vi "Transverse Triangulation Function.vi"(9 "output selector":T1, 10 "data":T2, 11 "X":dbl[](array[numeric])) -> (0 "error out":errorcluster, 1 "inequality constraint function values":dbl[](array[numeric]), 2 "equality constraint function values":dbl[](array[numeric]), 3 "objective function value":dbl)   [LabVIEW 2012]
doc: "This template is the starting point for creating an objective function, equality constraint function and inequality constraint function to be passed to the Constrained Nonlinear Optimization.vi."
uses:
  <vilib>/gmath/NumericalOptimization/objective function data.ctl
  <vilib>/gmath/NumericalOptimization/cno_output select.ctl
  <vilib>/gmath/NI_Gmath.lvlib
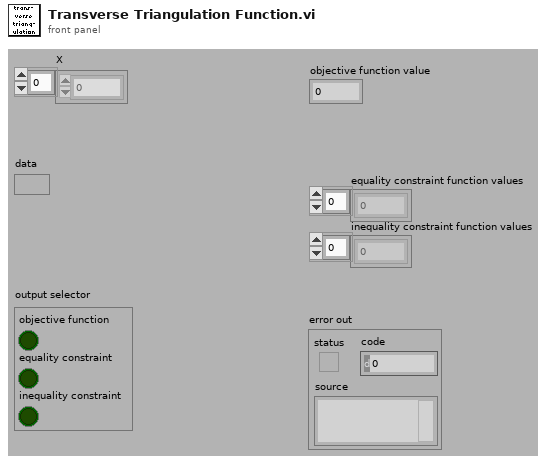
[diagram p1: front panel]
types:
  T1 = typedef "NI_Gmath.lvlib/cno_output select.ctl" = cluster{"objective function":bool, "equality constraint":bool, "inequality constraint":bool}
  T2 = typedef "NI_Gmath.lvlib/objective function data.ctl" = variant
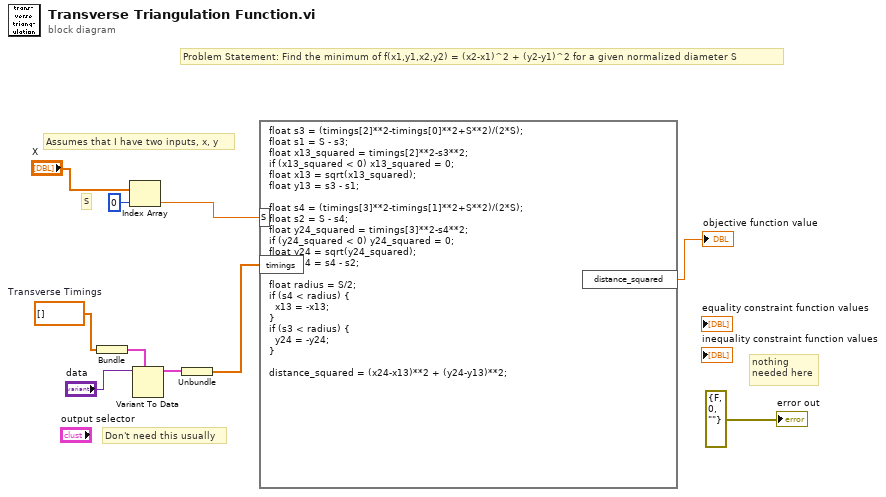
[diagram p0: block diagram]
diagram:
  w7 = dbl[] []  # Transverse Timings
  # "nothing \nneeded here"
  # "S"
  # "Problem Statement: Find the minimum of f(x1,y1,x2,y2) = (x2-x1)^2 + (y2-y1)^2 for a given normalized diameter S"
  # "Don't need this usually"
  # "Assumes that I have two inputs, x, y"
  n1 = Bundle("Transverse Timings"=w7) -> (w5:cluster{"Transverse Timings":dbl[]})  [unwired: 1 in]
  n2 = Index Array(array="X", index=0) -> (element=w2:dbl)
  n3 = Variant To Data(type=w5, Variant="data") -> (data=w4:cluster{"Transverse Timings":dbl[]})  [unwired: 1 in, 1 out]
  n4 = Unbundle(w4) -> ("Transverse Timings"=w3:dbl[])
  n5 = formula code="float s3 = (timings[2]**2-timings[0]**2+S**2)/(2*S);\nfloat s1 = S - s3;\nfloat x13_squared = timings[2]**2-s3**2;\nif (x13_squared < 0) x13_squared = 0;\nfloat x13 = sqrt(x13_squared);\nfloat y13 = s3 - s1;\n\nfloat s4 = (timings[3]**2-timings[1]**2+S**2)/(2*S);\nfloat s2 = S - s4;\nfloat y24_squared = timings[3]**2-s4**2;\nif (y24_squared < 0) y24_squared = 0;\nfloat y24 = sqrt(y24_squared);\nfloat x24 = s4 - s2;\n\nfloat radius = S/2;\nif (s4 < radius) {\n  x13 = -x13;\n}\nif (s3 < radius) {\n  y24 = -y24;\n}\n\ndistance_squared = (x24-x13)**2 + (y24-y13)**2;"("S"=w2, "timings"=w3) -> ("distance_squared"=→"objective function value":dbl)
  "error out" <- errorcluster {"status"=FALSE, "code"=0, "source"=""} ("error out")
